vi "fill_string2longs.vi"(11 "string_in":string) -> (3 "string_out":string)   [LabVIEW 2018]
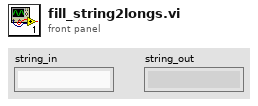
[diagram p1: front panel]
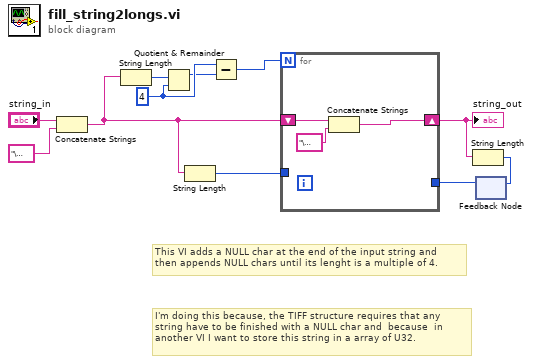
[diagram p0: block diagram]
diagram:
  w8 = 4 ("y")
  # "I'm doing this because, the TIFF structure requires that any string have to be finished with a NULL char and  because  in another VI I want to store this string in a array of U32."
  # "This VI adds a NULL char at the end of the input string and \nthen appends NULL chars until its lenght is a multiple of 4."
  n1 = Concatenate Strings("string_in", "\u0000") -> (w5:string)
  n2 = String Length(string=w5) -> (length=w6:i32)
  n3 = Quotient & Remainder(x=w6, y=w8) -> (x-y*floor(x/y)=w7:i32)  [unwired: 1 out]
  n4 = String Length(string=w5) -> (length=w4:i32)
  n5 = Subtract(x=w8, y=w7) -> (x-y=w9:i32)
  n6 = feedback #1() -> (w1:i32)  [unwired: 1 in]
  n7 = for {
    N: w9 -> [_]
    shift-right: [w14] -> w3
    shift-left: w5 -> [w13]
    tunnel: w4 -> [_]
    tunnel: w1 -> [_]
    n8 = Concatenate Strings(w13, "\u0000") -> (w14:string)
  }
  "string_out" <- w3
  n9 = String Length(string=w3) -> (length=w2:i32)
  n10 = feedback-in #1(w2) -> ()
